vi "Configure Statistics.vi"(7 "Statistical Type (0: Maximum Value)":i32(ring) items=["Maximum Value", "Minimum Value", "Mean Value", "Standard Deviation"], 8 "error in (no error)":errorcluster, 9 "Sample Size for Statistics (100)":i32=100, 10 "Statistics State (T: On)":bool=TRUE, 11 "VISA resource name":refnum<visa-resource-name>) -> (0 "error out":errorcluster, 3 "VISA resource name out":refnum<visa-resource-name>)   [LabVIEW 2019, in "Pendulum CNT90.lvlib"]
doc: "Configures statistical function. Switches On/Off the statistical function and selects the statistical function and sets the number of samples to use in statistics sampling."
uses:
  Pendulum CNT90.lvlib
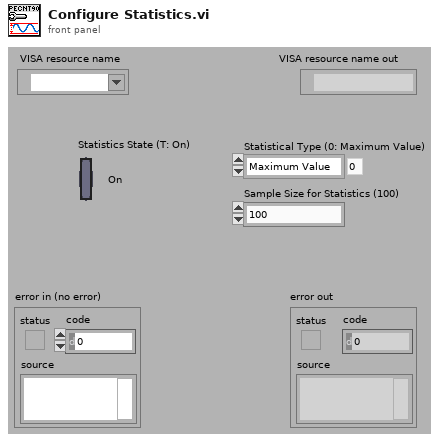
[diagram p1: front panel]
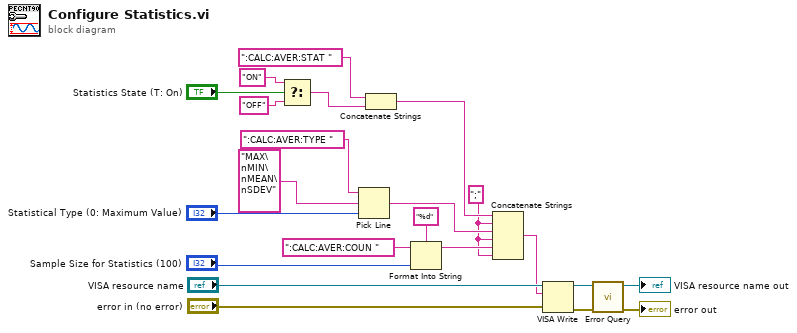
[diagram p0: block diagram]
diagram:
  w1 = ";" ("string")
  n1 = Select(t="ON", s="Statistics State (T: On)", f="OFF") -> (s? t:f=w12:string)
  n2 = Pick Line(string ("")=":CALC:AVER:TYPE ", multi-line string="MAX\nMIN\nMEAN\nSDEV", line index="Statistical Type (0: Maximum Value)") -> (output string=w7:string)
  n3 = Concatenate Strings(":CALC:AVER:STAT ", w12) -> (w8:string)
  n4 = Format Into String(format string="%d", initial string=":CALC:AVER:COUN " ("format string"), "Sample Size for Statistics (100)") -> (resulting string=w2:string)  [unwired: 1 in, 1 out]
  n5 = Concatenate Strings(w8, w1, w7, w1, w2, w1) -> (w6:string)
  n6 = VISA Write(VISA resource name="VISA resource name", write buffer=w6, error in (no error)="error in (no error)") -> (VISA resource name out=w20:refnum<visa-resource-name>, error out=w17:errorcluster)  [unwired: 1 out]
  n7 = call "Error Query.vi"("error in (no error)"=w17, "VISA resource name"=w20) -> ("error out"=→"error out":errorcluster, "VISA resource name out"=→"VISA resource name out":refnum<visa-resource-name>)  [unwired: 6 in, 2 out]
